vi "LVFunction_Imop_SlopesCompute_ModalZonalWavefront.vi"(0 "ModalCoef":refnum<class "ModalCoef.lvclass">, 1 "ComputePhaseSet":refnum<class "ComputePhaseSet.lvclass">, 2 "HasoSlopes":refnum<class "HasoSlopes.lvclass">, 5 "ResidualHasoSlopes":refnum<class "HasoSlopes.lvclass">, 7 "Phase":refnum<class "Phase.lvclass">, 11 "error constant":errorcluster) -> (4 "ModalCoef (dup)":refnum<class "ModalCoef.lvclass">, 6 "ResidualHasoSlopes (dup)":refnum<class "HasoSlopes.lvclass">, 8 "Phase (dup)":refnum<class "Phase.lvclass">, 15 "error out":errorcluster)   [LabVIEW 2020]
doc: "Compute phase from slopes using both zonal and modal reconstruction.\n\n--------------------------------------------------------------------------------\n\nHasoDataIn\n HasoData object.\n\nHasoDataOut\n HasoData object.\n\nComputePhaseSet\n cComputePhaseSet object.\n\nphaseC\n cPhase object.\n\nHasoSlopes\n cHasoSlopes object containing the residual slopes.\n\nErrorIn\n Error\nErrorOut\n Error"
uses:
  ComputePhaseSet.lvclass
  HasoSlopes.lvclass
  Phase.lvclass
  ModalCoef.lvclass
  LVClass_ModalCoef Read ModalCoef.vi
  LVClass_HasoSlopes Read HasoSlopes _ property.vi
  LVClasse_Phase Read SurfaceFloatWithPupil.vi
  LVClass_ComputePhaseSet Read ComputePhaseSet.vi
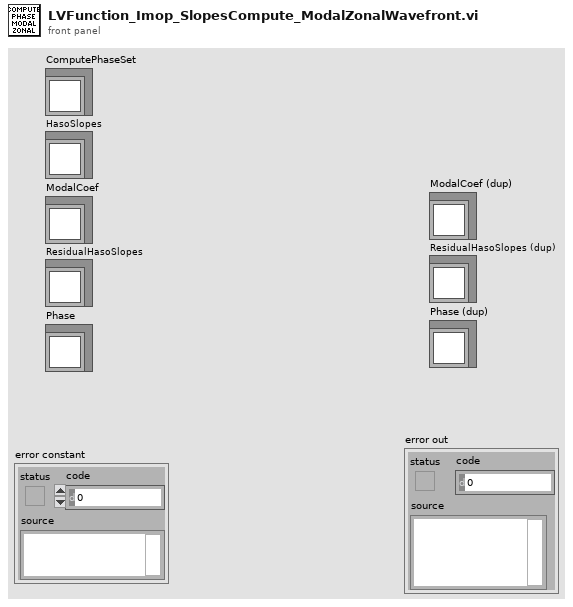
[diagram p1: front panel]
types:
  T1 = typedef "ClassID.ctl" = i64
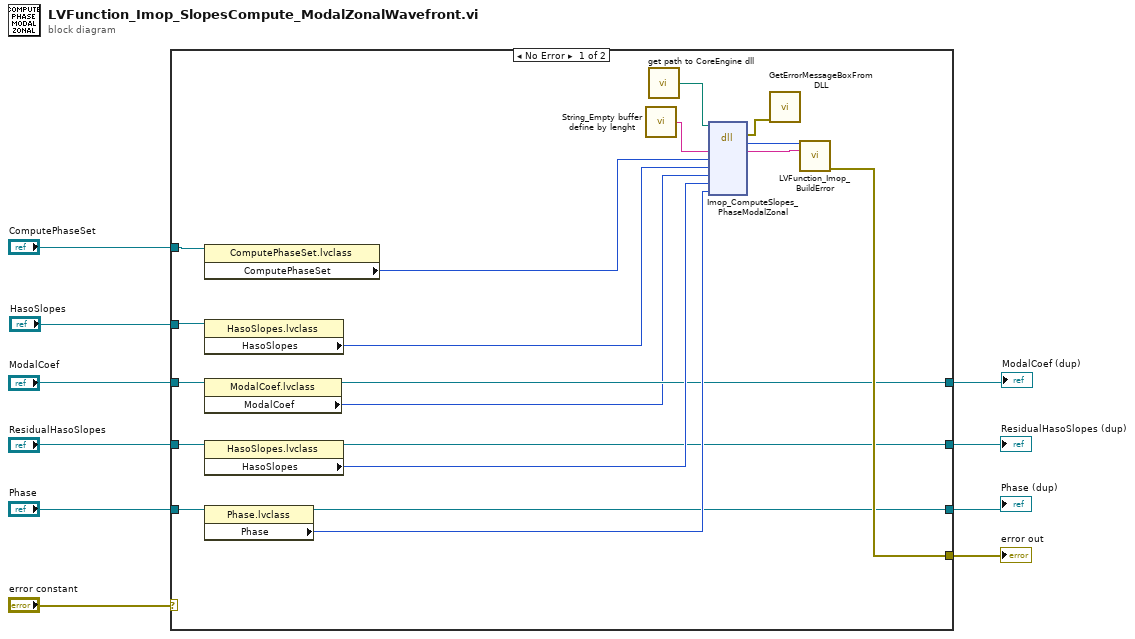
[diagram p0: block diagram]
diagram:
  n1 = case shown="No Error" "error constant" {
    selector: "error constant" -> [_ w33]
    tunnel: "HasoSlopes" -> [w23 _]
    tunnel: "ComputePhaseSet" -> [w22 _]
    tunnel: [w24 w33] -> w9
    tunnel: "Phase" -> [w21 w32]
    tunnel: "ResidualHasoSlopes" -> [w17 w31]
    tunnel: [w15 w32] -> w6
    tunnel: [w14 w31] -> w4
    tunnel: "ModalCoef" -> [w13 w30]
    tunnel: [w12 w30] -> w2
    frame No Error {
      n2 = property class="ComputePhaseSet.lvclass"(reference=w22) -> ("ComputePhaseSet"=w19:T1)  [unwired: 1 in, 2 out]
      n3 = property class="HasoSlopes.lvclass"(reference=w23) -> ("HasoSlopes"=w20:T1)  [unwired: 1 in, 2 out]
      n4 = property class="ModalCoef.lvclass"(reference=w13) -> (reference out=w12:refnum<class "ModalCoef.lvclass">, "ModalCoef"=w11:T1)  [unwired: 1 in, 1 out]
      n5 = property class="HasoSlopes.lvclass"(reference=w17) -> (reference out=w14:refnum<class "HasoSlopes.lvclass">, "HasoSlopes"=w16:T1)  [unwired: 1 in, 1 out]
      n6 = property class="Phase.lvclass"(reference=w21) -> (reference out=w15:refnum<class "Phase.lvclass">, "Phase"=w18:T1)  [unwired: 1 in, 1 out]
      n7 = call "String_Empty buffer define by lenght.vi"() -> ("Empty buffer"=w27:string)  [unwired: 1 in]
      n8 = call "get path to CoreEngine dll.vi"() -> ("path to wavekit library"=w26:path)  [unwired: 14 in, 1 out]
      n9 = dll-call lib="D:/FLE/0.Code/CoreEngine4_Suite/LV2011_interface/DLLs/c_interface_vc100.dll" fn="Imop_ComputeSlopes_PhaseModalZonal"(path in=w26, "message"=w27, "ComputePhaseSet"=w19, "HasoSlopes"=w20, "ModalCoeffs"=w11, "ResidualHasoSlopes"=w16, "Phase"=w18) -> (error out=w25:errorcluster, "return type"=w29:i32, "message"=w28:string)  [unwired: 7 in, 1 out]
      n10 = call "GetErrorMessageBoxFromDLL.vi"("error IN"=w25) -> ()  [unwired: 10 in, 1 out]
      n11 = call "LVFunction_Imop_BuildError.vi"("code"=w29, "String to Prepend to source (\"\")"=w28) -> ("error out"=w24:errorcluster)  [unwired: 13 in]
    }
    frame Error {
    }
  }
  "error out" <- w9
  "Phase (dup)" <- w6
  "ResidualHasoSlopes (dup)" <- w4
  "ModalCoef (dup)" <- w2
